vi "Windows Title.vi"(8 "error in (no error)":errorcluster, 9 "Data":string, 10 "ActorQName":string, 11 "UI_Top in":refnum<class "UI_Top.lvclass">) -> (0 "error out":errorcluster, 3 "UI_Top out":refnum<class "UI_Top.lvclass">)   [LabVIEW 2021, in "UI_Top.lvclass"]
uses:
  UI_Top.lvclass
  UI_Top.lvclass/UI_Top.ctl
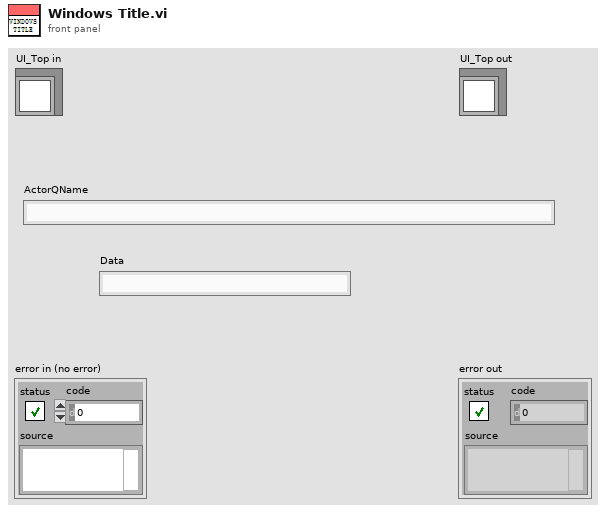
[diagram p1: front panel]
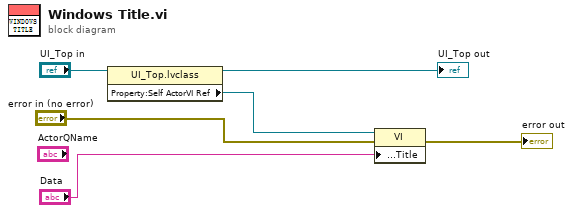
[diagram p0: block diagram]
diagram:
  n1 = property class="UI_Top.lvclass"(reference="UI_Top in") -> (reference out=→"UI_Top out":refnum<class "UI_Top.lvclass">, "Property:Self ActorVI Ref"=w4:refnum<vi>)  [unwired: 1 in, 1 out]
  n2 = property class="VI"(reference=w4, error in="error in (no error)", "Front Panel.Title"="Data") -> (error out=→"error out":errorcluster)  [unwired: 1 out]
